vi "TestLakeshore218.vi"() -> ()   [LabVIEW 2018]
panel:
  out "Thick Film R (Ohms)":string
  out "Level Resistor (Low)":dbl
  out "Level Resistor (High)":dbl
  out "error out":errorcluster
  in  "Stop":bool
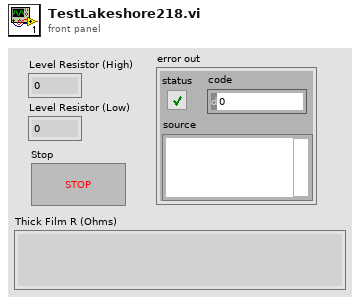
[diagram p1: front panel]
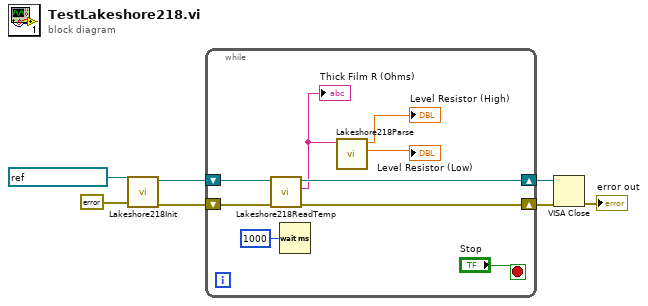
[diagram p0: block diagram]
diagram:
  n1 = call "Lakeshore218Init.vi"("error in (no error)"=errorcluster {"status"=FALSE, "code"=0, "source"=""}, "VISA resource name"=refnum<visa-resource-name> "Lakeshore218") -> ("error out"=w5:errorcluster, "VISA resource name out"=w4:refnum<visa-resource-name>)  [unwired: 8 in]
  n2 = while {
    shift-right: [w13] -> w2
    shift-left: w4 -> [w14]
    shift-right: [w12] -> w3
    shift-left: w5 -> [w15]
    stop <- "Stop" stop-if-true
    n3 = call "Lakeshore218ReadTemp.vi"("error in"=w15, "VISA resource name"=w14) -> ("error out"=w12:errorcluster, "Thick Film R (Ohms)"=w10:string, "VISA resource name out"=w13:refnum<visa-resource-name>)  [unwired: 7 in]
    "Thick Film R (Ohms)" <- w10
    n4 = Wait (ms)(milliseconds to wait=u32 1000) -> ()  [unwired: 1 out]
    n5 = call "Lakeshore218Parse.vi"("Resistance String"=w10) -> ("Low Level (Ohms)"=→"Level Resistor (Low)":dbl, "High Level (Ohms)"=→"Level Resistor (High)":dbl)  [unwired: 9 in]
  }
  n6 = VISA Close(VISA resource name=w2, error in (no error)=w3) -> (error out=→"error out":errorcluster)
